vi "Constructor.vi"() -> (3 "data value reference":T1)   [LabVIEW 2016, in "Impulse Data.lvclass"]
uses:
  Impulse Data.lvclass
  Instance handle.ctl
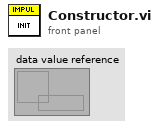
[diagram p1: front panel]
types:
  T1 = typedef "Impulse Data.lvclass/Instance handle.ctl" = refnum<data-value>
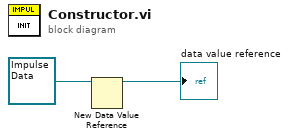
[diagram p0: block diagram]
diagram:
  n1 = New Data Value Reference(data value=refnum<class "Impulse Data.lvclass"> refnum ("Impulse Data.lvclass")) -> (data value reference=→"data value reference":refnum<data-value>)  [unwired: 1 in, 1 out]
